vi "Send Get Device Parameter Status.vi"(4 "Parameter/Error":string, 5 "Get Device Parameter Status Msg":refnum<class "Get Device Parameter Status Msg.lvclass">, 6 "Status":T2, 7 "Message Priority (Normal)":T1=enum."Normal", 8 "error in (no error)":errorcluster, 9 "Parameter Name":string, 10 "IED Name":string, 11 "Message Enqueuer in":refnum<class "Message Enqueuer.lvclass">) -> (0 "error out":errorcluster, 3 "Message Enqueuer out":refnum<class "Message Enqueuer.lvclass">)   [LabVIEW 2015, in "SCADA Core.lvlib" / "Get Device Parameter Status Msg.lvclass"]
uses:
  Get Device Parameter Status Msg.lvclass
  Get Device Parameter Status.ctl
  <vilib>/ActorFramework/Message Enqueuer/Message Enqueuer.lvclass
  <vilib>/ActorFramework/Message Enqueuer/Message Priority.ctl
  Get Device Parameter Status Msg.lvclass/Get Device Parameter Status Msg.ctl
  <vilib>/ActorFramework/Message Enqueuer/Message Enqueuer.lvclass/Message Enqueuer.ctl
  <vilib>/ActorFramework/Message Priority Queue/Priority Enqueue.vi
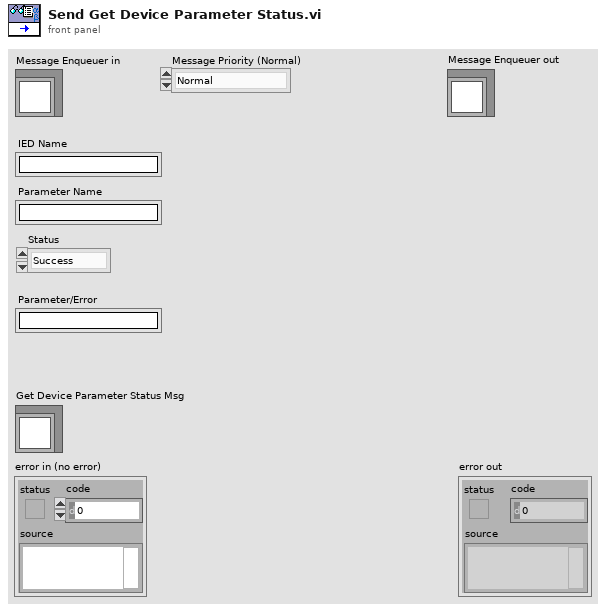
[diagram p1: front panel]
types:
  T1 = typedef "Actor Framework.lvlib/Message Enqueuer.lvclass/Message Priority.ctl" = enum16{"Low", "Normal", "High"}
  T2 = typedef "SCADA Core.lvlib/Get Device Parameter Status Msg.lvclass/Get Device Parameter Status.ctl" = enum16{"Success", "Failure"}
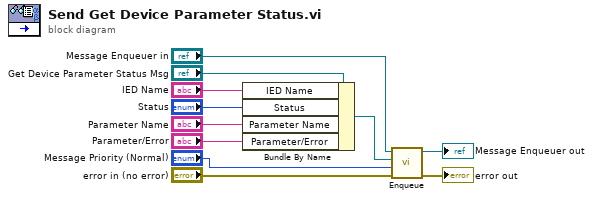
[diagram p0: block diagram]
diagram:
  n1 = Bundle By Name(cluster="Get Device Parameter Status Msg", "IED Name"="IED Name", "Status"="Status", "Parameter Name"="Parameter Name", "Parameter/Error"="Parameter/Error") -> (w5:refnum<class "Get Device Parameter Status Msg.lvclass">)
  n2 = call <vilib>:"Enqueue.vi"("error in (no error)"="error in (no error)", "Message Priority (Normal)"="Message Priority (Normal)", "Message"=w5, "Message Enqueuer in"="Message Enqueuer in") -> ("error out"=→"error out":errorcluster, "Message Enqueuer out"=→"Message Enqueuer out":refnum<class "Message Enqueuer.lvclass">)  [unwired: 6 in]
